vi "ep13_while_loop.vi"() -> ()   [LabVIEW 2019]
panel:
  out "x+y":i32
  out "number: 0 to 1":dbl
  out "Array 2":dbl[](array[numeric])
  out "Array":dbl[](array[numeric])
  out "Numeric":i32
  in  "stop":bool
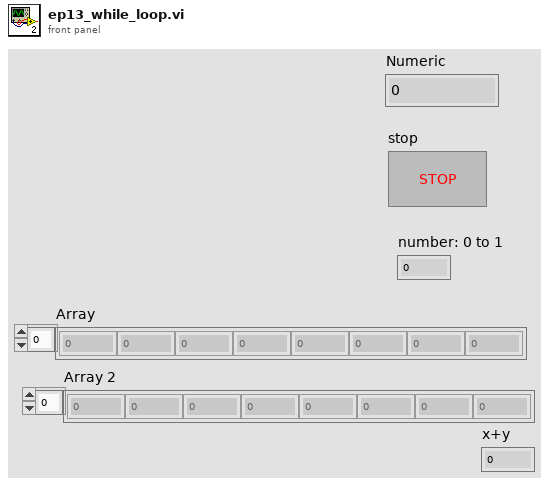
[diagram p1: front panel]
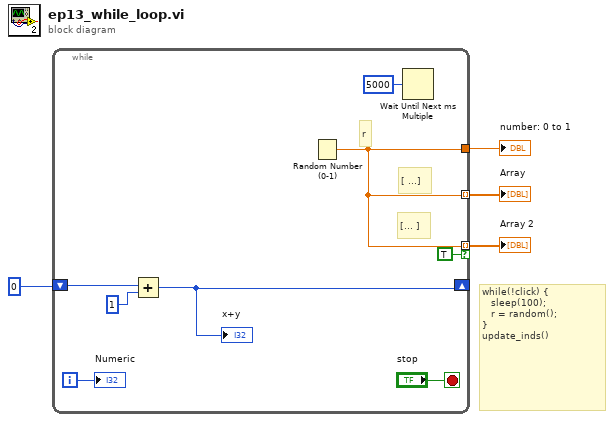
[diagram p0: block diagram]
diagram:
  # "while(!click) {\n   sleep(100);\n   r = random();\n}\nupdate_inds()"
  n1 = while {
    tunnel: [w10] -> w2
    tunnel: [w10] -> w4 mode=indexing
    tunnel: [w10] -> w3 mode=indexing if=TRUE
    shift-right: [w5] -> _
    shift-left: 0 -> [w7]
    i -> [w8]
    stop <- "stop" stop-if-true
    # "[... ]"
    # "[ ...]"
    # "r"
    n2 = Add(x=w7, y=1) -> (x+y=w5:i32)
    "x+y" <- w5
    n3 = Random Number (0-1)() -> (number: 0 to 1=w10:dbl)
    n4 = Wait Until Next ms Multiple(millisecond multiple=u32 5000) -> ()  [unwired: 1 out]
    "Numeric" <- w8
  }
  "Array" <- w4
  "Array 2" <- w3
  "number: 0 to 1" <- w2
